vi "Error-Status.vi"(3 "error in (no error)":errorcluster) -> (1 "Boolean":bool)   [LabVIEW 2020]
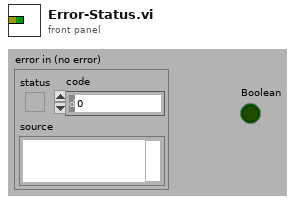
[diagram p1: front panel]
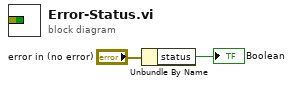
[diagram p0: block diagram]
diagram:
  n1 = Unbundle By Name("error in (no error)") -> ("status"=→"Boolean":bool)
